vi "pf_Get_3D-COP.vi"(0 "IMAQ Session in":refnum<k11>, 1 "Truncate Range":bool, 5 "Range Map in":sgl[][](array[numeric]), 7 "Range Max":sgl=1024.0, 9 "Range Min":sgl, 11 "error in (no error)":errorcluster, 12 "dx":sgl=1.0, 13 "dy":sgl=1.0) -> (4 "IMAQ Session out":refnum<k11>, 6 "X Matrix":sgl[][](array[numeric]), 8 "Y Matrix":sgl[][](array[numeric]), 10 "Z Matrix":sgl[][](array[numeric]), 15 "error out":errorcluster)   [LabVIEW 2012, in "Photonfocus_Toolkit.lvlib"]
doc: "Gets a 3D Cloud of Points from a Range Map.\nThis VI is useful to plot 3D data (see related examples)."
uses:
  <userlib>/Photonfocus Toolkit/Photonfocus_Toolkit.lvlib
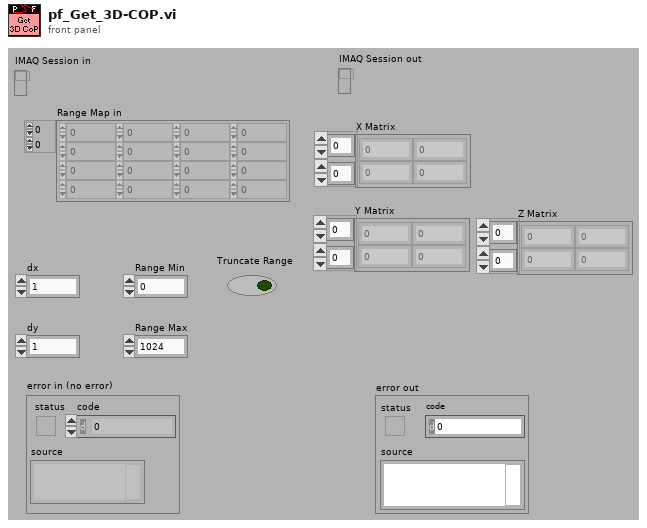
[diagram p1: front panel]
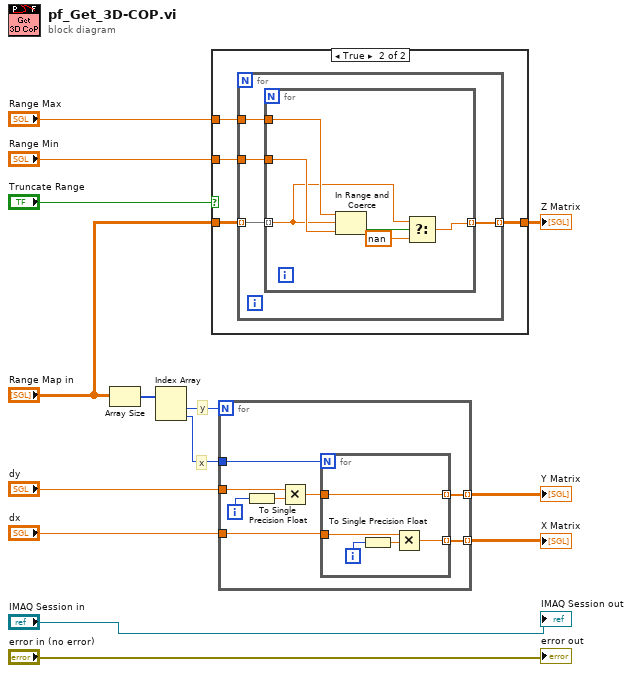
[diagram p0: block diagram]
diagram:
  # "x"
  # "y"
  n1 = Array Size(array="Range Map in") -> (size(s)=w14:i32[])
  n2 = Index Array(array=w14) -> (element #1=w13:i32, element #2=w10:i32)  [unwired: 2 in]
  n3 = case shown="True" "Truncate Range" {
    tunnel: "Range Map in" -> [w15 w19]
    tunnel: "Range Max" -> [_ w18]
    tunnel: "Range Min" -> [_ w17]
    tunnel: [w15 w16] -> w1
    frame False {
    }
    frame True {
      n4 = for {
        tunnel: w19 -> [w23] mode=indexing
        tunnel: w18 -> [w22]
        tunnel: w17 -> [w21]
        tunnel: [w20] -> w16 mode=indexing
        n5 = for {
          tunnel: w23 -> [w26] mode=indexing
          tunnel: w22 -> [w29]
          tunnel: w21 -> [w28]
          tunnel: [w24] -> w20 mode=indexing
          n6 = In Range and Coerce(upper limit=w29, x=w26, lower limit=w28) -> (In Range?=w27:bool)  [unwired: 1 out]
          n7 = Select(t=w26, s=w27, f=sgl nan) -> (s? t:f=w24:sgl)
        }
      }
    }
  }
  "Z Matrix" <- w1
  n8 = for {
    N: w13 -> [_]
    tunnel: "dy" -> [w37]
    tunnel: "dx" -> [w34]
    tunnel: w10 -> [w33]
    tunnel: [w31] -> w3 mode=indexing
    tunnel: [w30] -> w2 mode=indexing
    i -> [w36]
    n9 = To Single Precision Float(number=w36) -> (single precision float=w35:sgl)
    n10 = Multiply(x=w37, y=w35) -> (x*y=w32:sgl)
    n11 = for {
      N: w33 -> [_]
      tunnel: w34 -> [w42]
      tunnel: [w39] -> w30 mode=indexing
      tunnel: [w38] -> w31 mode=indexing
      tunnel: w32 -> [w38]
      i -> [w41]
      n12 = To Single Precision Float(number=w41) -> (single precision float=w40:sgl)
      n13 = Multiply(x=w42, y=w40) -> (x*y=w39:sgl)
    }
  }
  "Y Matrix" <- w3
  "X Matrix" <- w2
  "error out" <- "error in (no error)"
  "IMAQ Session out" <- "IMAQ Session in"
